vi "amazing script into vi.vi"(0 "Image In":T3, 7 "error in":errorcluster) -> (20 "Image Out":T3, 21 "Clamp Results (Max Clamp 1)":T2, 22 "Clamp Points (Max Clamp 1)":T1, 27 "error out":errorcluster)   [LabVIEW 2016]
uses:
  <vilib>/vision/Image Controls.llb/IMAQ Image.ctl
  <vilib>/vision/Pattern Matching.llb/IMAQ Curve Parameters.ctl
  <vilib>/vision/NI_Vision_Development_Module.lvlib
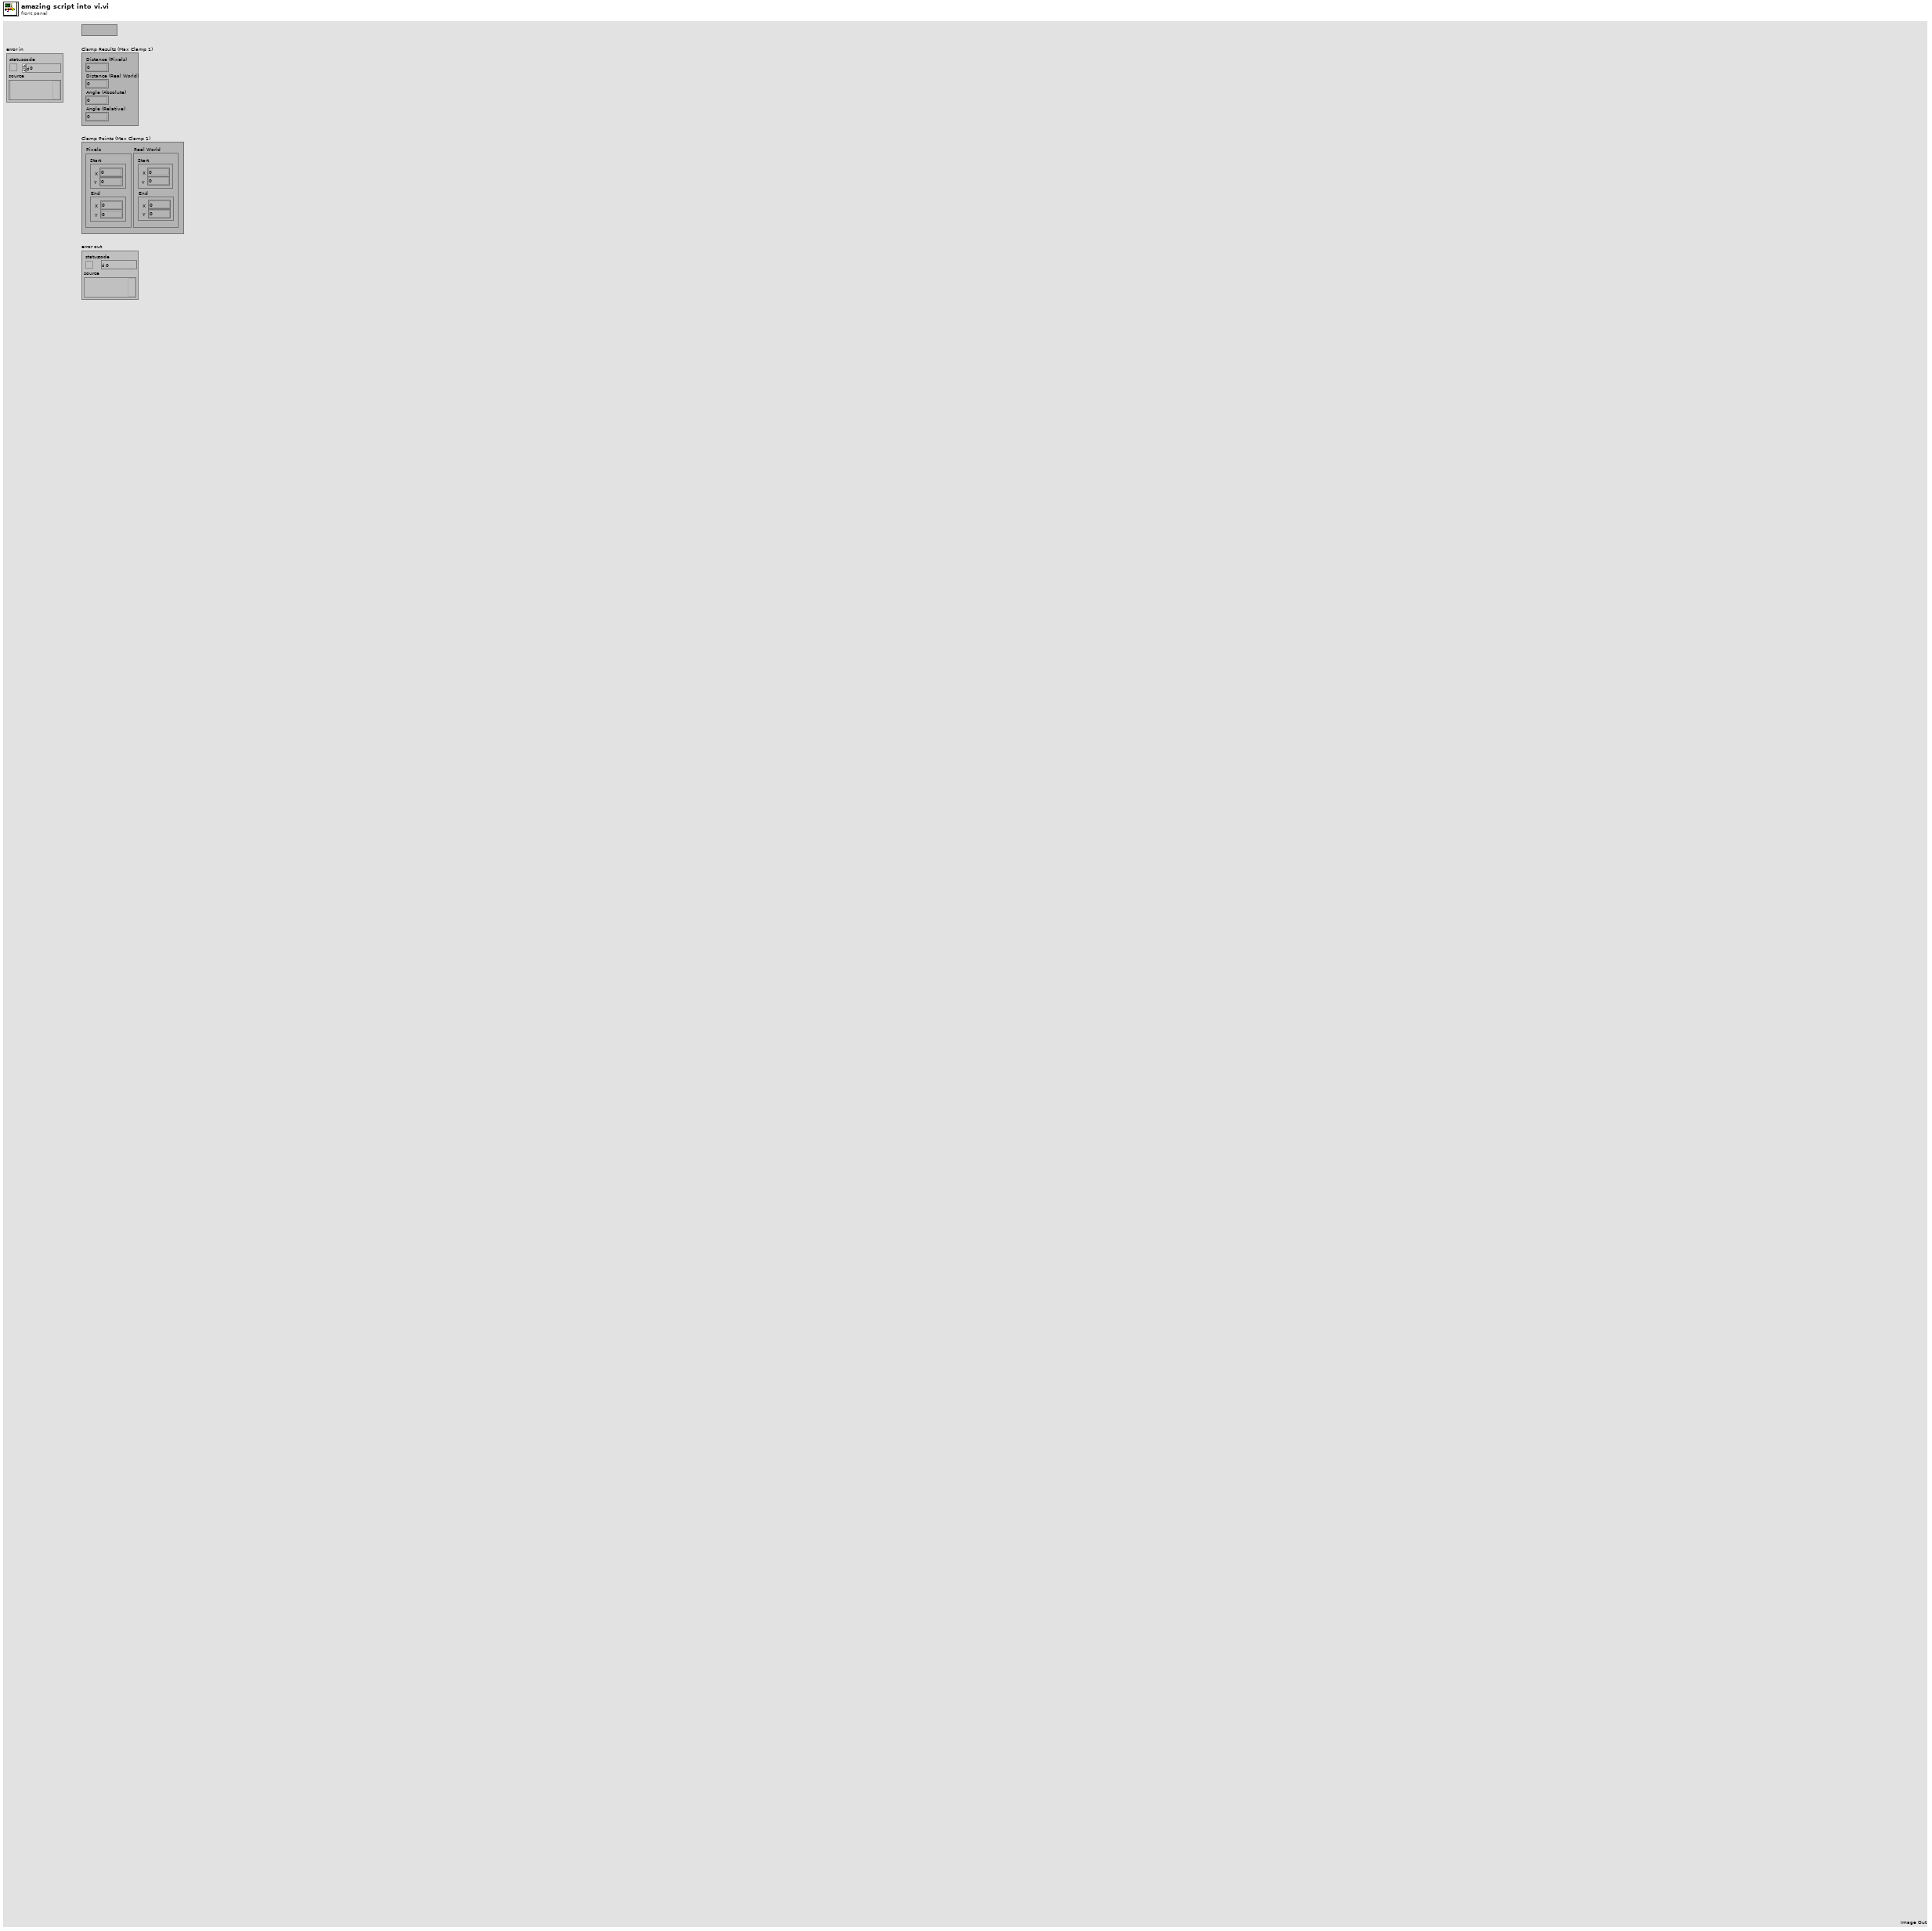
[diagram p1: front panel]
types:
  T1 = cluster{"Pixels ":cluster{"Start":cluster{"X":dbl, "Y":dbl}, "End":cluster{"X":dbl, "Y":dbl}}, "Real World":cluster{"Start":cluster{"X":dbl, "Y":dbl}, "End":cluster{"X":dbl, "Y":dbl}}}
  T2 = cluster{"Distance (Pixels)":dbl, "Distance (Real World)":dbl, "Angle (Absolute)":dbl, "Angle (Relative)":dbl}
  T3 = typedef "IMAQ Image.ctl" = refnum<image>
  T4 = cluster{"Angle Range (+/-)":dbl, "Edge Polarity":cluster{"Start":u32, "End":u32}}
  T5 = typedef "IMAQ Curve Parameters.ctl" = cluster{"Extraction Mode":u32, "Edge Threshold":i32, "Edge Filter Size":u32, "Min Length":i32, "Row Search Step Size":i32, "Col Search Step Size":i32, "Max Endpoint Gap":i32, "Closed":bool, "Subpixel":bool}
  T6 = cluster{"Show Search Area":bool, "Show Curves":bool, "Show Clamp Locations":bool, "Show Result":bool, "Search Area Color":u32, "Curves Color":u32, "Clamp Locations Color":u32, "Result Color":u32, "Overlay Group Name":string}
  T7 = cluster{"Global Rectangle":i32[], "Contours":cluster{"ID":enum32{"External", "Internal"}, "Type":u32, "Coordinates":i32[]}[]}
  T8 = enum32{"AutoM", "Close", "Dilate", "Erode", "Gradient", "Gradient in", "Gradient out", "HitMiss", "Open", "PClose", "POpen", "Thick", "Thin"}
  T9 = enum32{"Linear", "Log", "Exp", "Square", "Square root", "Power X", "Power 1/X"}
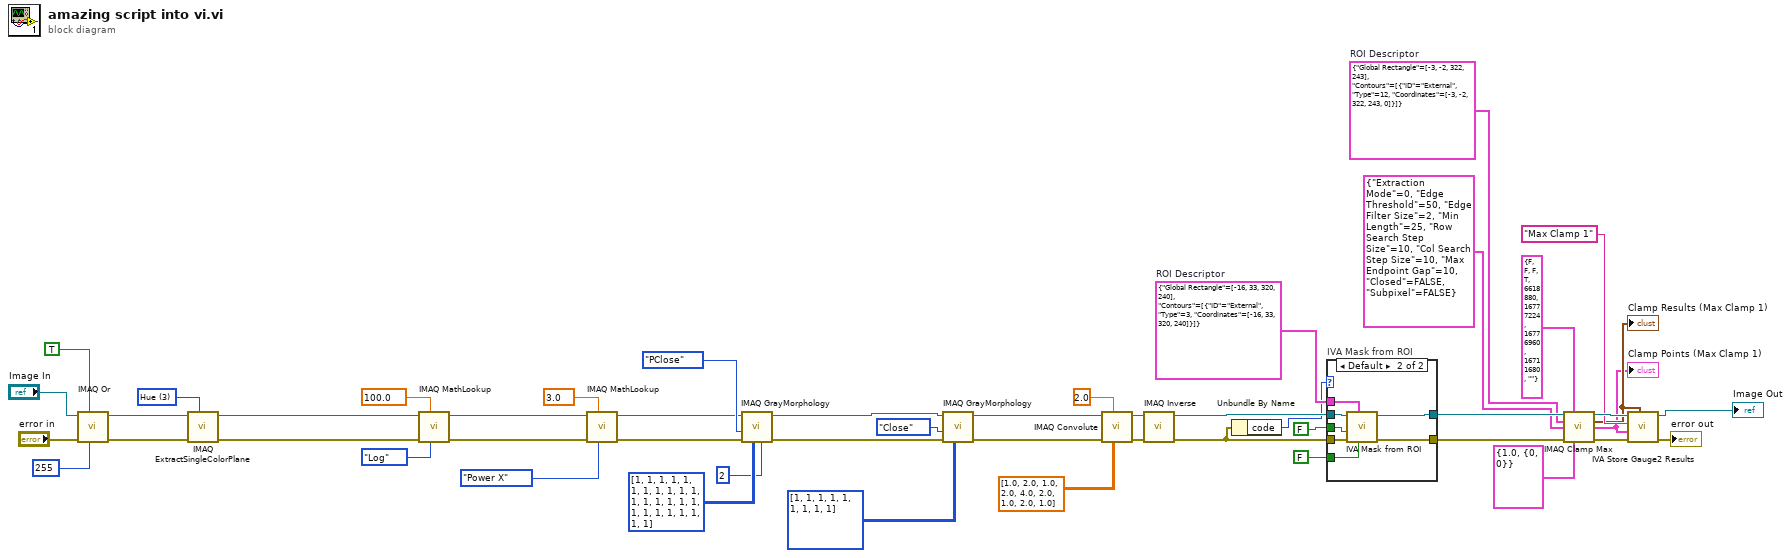
[diagram p0: block diagram]
diagram:
  w5 = T7 {"Global Rectangle"=[-3, -2, 322, 243], "Contours"=[{"ID"=enum."External", "Type"=12, "Coordinates"=[-3, -2, 322, 243, 0]}]}  # ROI Descriptor
  w19 = T7 {"Global Rectangle"=[-16, 33, 320, 240], "Contours"=[{"ID"=enum."External", "Type"=3, "Coordinates"=[-16, 33, 320, 240]}]}  # ROI Descriptor
  w45 = 3 items=["Red", "Green", "Blue", "Hue", "Saturation", "Luminance", "Value", "Intensity"] ("Color Plane")
  n1 = call "IMAQ Or"("Constant"=255, "Or/Nor (Or)"=TRUE, "error in (no error)"="error in", "Image Src A"="Image In") -> ("error out"=w43:errorcluster, "Image Dst Out"=w44:T3)  [unwired: 2 in, 4 out]
  n2 = call "IMAQ ExtractSingleColorPlane"("Color Plane"=w45, "error in (no error)"=w43, "Image Src"=w44) -> ("error out"=w39:errorcluster, "Image Dst Out"=w40:T3)  [unwired: 1 in, 6 out]
  n3 = call "IMAQ MathLookup"("Operator"=T9."Log", "X Value"=sgl 100.0, "error in (no error)"=w39, "Image Src"=w40) -> ("error out"=w35:errorcluster, "Image Dst Out"=w36:T3)  [unwired: 3 in, 3 out]
  n4 = call "IMAQ MathLookup"("Operator"=T9."Power X", "X Value"=sgl 3.0, "error in (no error)"=w35, "Image Src"=w36) -> ("error out"=w31:errorcluster, "Image Dst Out"=w32:T3)  [unwired: 3 in, 3 out]
  n5 = call "IMAQ GrayMorphology"("Number of iterations (1)"=2, "Structuring Element"=i32[][] [[1, 1, 1, 1, 1], [1, 1, 1, 1, 1], [1, 1, 1, 1, 1], [1, 1, 1, 1, 1], [1, 1, 1, 1, 1]], "error in (no error)"=w31, "Operation"=T8."PClose", "Image Src"=w32) -> ("error out"=w26:errorcluster, "Image Dst Out"=w27:T3)  [unwired: 2 in, 3 out]
  n6 = call "IMAQ GrayMorphology"("Structuring Element"=i32[][] [[1, 1, 1], [1, 1, 1], [1, 1, 1]], "error in (no error)"=w26, "Operation"=T8."Close", "Image Src"=w27) -> ("error out"=w23:errorcluster, "Image Dst Out"=w24:T3)  [unwired: 3 in, 3 out]
  n7 = call "IMAQ Convolute"("Kernel"=sgl[][] [[1.0, 2.0, 1.0], [2.0, 4.0, 2.0], [1.0, 2.0, 1.0]], "Divider (kernel sum)"=sgl 2.0 ("Divider"), "error in (no error)"=w23, "Image Src"=w24) -> ("error out"=w20:errorcluster, "Image Dst Out"=w21:T3)  [unwired: 3 in, 3 out]
  n8 = call "IMAQ Inverse"("error in (no error)"=w20, "Image Src"=w21) -> ("error out"=w15:errorcluster, "Image Dst Out"=w17:T3)  [unwired: 2 in, 6 out]
  n9 = Unbundle By Name(w15) -> ("code"=w14:i32)
  n10 = case "IVA Mask from ROI" shown="Default" w14 {
    tunnel: w19 -> [_ w57]
    tunnel: FALSE ("Shrink") -> [_ w56]
    tunnel: w17 -> [w50 w55]
    tunnel: w15 -> [_ w54]
    tunnel: [_ w53] -> w11
    tunnel: [w50 w52] -> w12
    tunnel: FALSE ("Out / In") -> [_ w51]
    frame -1074396199, -1074396198 {
      # "Discard\nCoordinate\nSystem\nError"
    }
    frame Default {
      n11 = call <vilib>:"IVA Mask from ROI.vi"("Shrink"=w56, "ROI Descriptor"=w57, "error in (no error)"=w54, "Out / In"=w51, "Image Src"=w55) -> ("error out"=w53:errorcluster, "Image Out"=w52:T3)  [unwired: 5 out]
    }
  }
  n12 = call "IMAQ Clamp Max"("Source Image"=w12, "Overlay Settings"=T6 {"Show Search Area"=FALSE, "Show Curves"=FALSE, "Show Clamp Locations"=FALSE, "Show Result"=TRUE, "Search Area Color"=6618880, "Curves Color"=16777224, "Clamp Locations Color"=16776960, "Result Color"=16711680, "Overlay Group Name"=""}, "ROI Descriptor"=w5, "Curve Extraction Settings"=T5 {"Extraction Mode"=0, "Edge Threshold"=50, "Edge Filter Size"=2, "Min Length"=25, "Row Search Step Size"=10, "Col Search Step Size"=10, "Max Endpoint Gap"=10, "Closed"=FALSE, "Subpixel"=FALSE}, "error in (no error)"=w11, "Clamp Settings"=T4 {"Angle Range (+/-)"=1.0, "Edge Polarity"={"Start"=0, "End"=0}}) -> ("Image Out"=w10:T3, "Clamp Results"=w2:T2, "Clamp Points"=w1:T1, "error out"=w13:errorcluster)  [unwired: 1 in, 5 out]
  "Clamp Results (Max Clamp 1)" <- w2
  "Clamp Points (Max Clamp 1)" <- w1
  n13 = call <vilib>:"IVA Store Gauge2 Results.vi"("Clamp Results"=w2, "error in (no error)"=w13, "Clamp Points"=w1, "Step Name"="Max Clamp 1", "Image in"=w10) -> ("error out"=→"error out":errorcluster, "Image Out"=→"Image Out":T3)  [unwired: 5 out]
